vi "Check_int_points_allowed.vi"(11 "Integration Points":dbl) -> (0 "Output Integration":dbl, 3 "String":string)   [LabVIEW 2021]
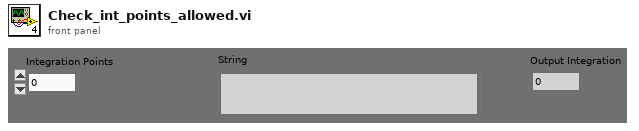
[diagram p1: front panel]
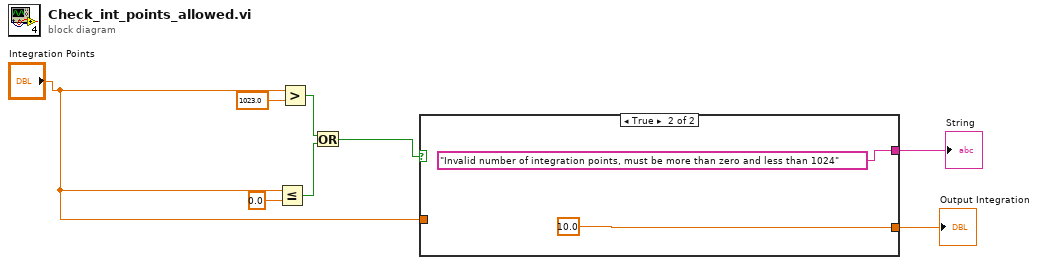
[diagram p0: block diagram]
diagram:
  n1 = Less Or Equal?(x="Integration Points", y=0.0) -> (x <= y?=w6:bool)
  n2 = Greater?(x="Integration Points", y=1023.0) -> (0:w1:bool)
  n3 = Or(x=w1, y=w6) -> (x .or. y?=w5:bool)
  n4 = case shown="True" w5 {
    tunnel: [_ "Invalid number of integration points, must be more than zero and less than 1024"] -> w4
    tunnel: "Integration Points" -> [w9 _]
    tunnel: [w9 10.0 ("Integration Points")] -> w2
    frame False {
    }
    frame True {
    }
  }
  "String" <- w4
  "Output Integration" <- w2
